vi "Main.Get Compiled Settings.vi"(8 "error in (no error)":errorcluster, 11 "Item Ref in":T1 format="%.0x") -> (0 "error out":errorcluster, 3 "Compiled":T2 {"Nodes"."Monitor"."Network"."Name" format="%.0x"; "Nodes"."Sim"."Network"."Name" format="%.0x"; "XNET"."Termination" items=["Off", "On"]})   [LabVIEW 2019, in "J1939 Addon Engine.lvlib"]
uses:
  J1939 Addon Engine.lvlib
  Addon Shared/Types/Compile Addon Settings.ctl
  Addon Shared/Types/XNET Settings.ctl
  Addon Shared/Types/SysDef FPGA Settings.ctl
  Addon Shared/Types/Compiled.Node Settings.ctl
  Addon Shared/Types/Compiled Monitor Tool Settings.ctl
  Addon Shared/Types/Monitor Settings.ctl
  Addon Shared/Types/Device Settings.ctl
  Addon Shared/Types/Incoming Settings.ctl
  Addon Shared/Types/Incoming Frame Settings.ctl
  <vilib>/NI VeriStand/Custom Device API/Block Data Reference.ctl
  <vilib>/NI VeriStand/Custom Device API/Data Reference.ctl
  Addon Shared/Types/Outgoing Settings.ctl
  Addon Shared/Types/Outgoing Frame Settings.ctl
  Addon Shared/Types/Outgoing Event Trigger Types.ctl
  SubModules/Frame-Protection-Support/Source/Shared/Types/Exported Frame Settings.ctl
  SubModules/Frame-Protection-Support/Source/Shared/Types/Exported Frame Type.ctl
  SubModules/Frame-Protection-Support/Source/Shared/Types/Exported Protection Settings.ctl
  SubModules/Frame-Protection-Support/Source/Shared/Types/Protection Type.ctl
  SubModules/Frame-Protection-Support/Source/Shared/Types/XNET Signal Configuration.ctl
  SubModules/Frame-Protection-Support/Source/Shared/Types/Exported Counter Settings.ctl
  SubModules/Frame-Protection-Support/Source/Shared/Types/Exported Event Trigger Type.ctl
  Addon Shared/Types/Complied Simulated Device Settings.ctl
  Addon Shared/Types/Compiled Simulated Settings.ctl
  <vilib>/NI VeriStand/Custom Device API/Custom Device Item Ref.ctl
  Addon Shared/SubVIs/Constants.vi
  <vilib>/NI VeriStand/Custom Device API/Get Item Property (Variant).vi
  <vilib>/NI VeriStand/Custom Device API/Custom Device API.lvlib
  Addon Shared/J1939 Addon Shared.lvlib
  SubModules/Frame-Protection-Support/Source/Shared/Protection and Counter Support Shared.lvlib
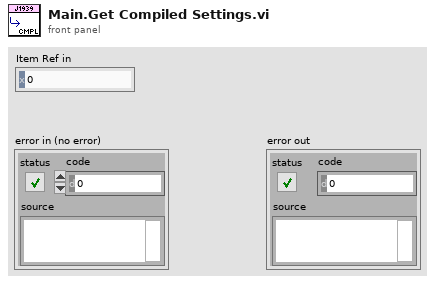
[diagram p1: front panel]
types:
  T1 = typedef "Custom Device API.lvlib/Custom Device Item Ref.ctl" = u64
  T2 = typedef "J1939 Addon Shared.lvlib/Compile Addon Settings.ctl" = cluster{"XNET":T3, "Bitfile":T4, "Nodes":T5, "Name":string}
  T3 = typedef "J1939 Addon Shared.lvlib/XNET Settings.ctl" = cluster{"Database":refnum<k21>, "Cluster":refnum<k21>, "Port":string, "Baud rate [Bd]":u32, "Termination":u32, "Incoming Decimation":u32, "Outgoing Decimation":u32}
  T4 = typedef "J1939 Addon Shared.lvlib/SysDef FPGA Settings.ctl" = cluster{"RT Path":path, "RIO Device":string, "Enable":bool}
  T5 = typedef "J1939 Addon Shared.lvlib/Compiled.Node Settings.ctl" = cluster{"Monitor":T6, "Sim":T23[]}
  T6 = typedef "J1939 Addon Shared.lvlib/Compiled Monitor Tool Settings.ctl" = cluster{"Network":T7, "Data":T8}
  T7 = typedef "J1939 Addon Shared.lvlib/Monitor Settings.ctl" = cluster{"Address":u8, "Name":u64, "Include DA":bool}
  T8 = typedef "J1939 Addon Shared.lvlib/Device Settings.ctl" = cluster{"Incoming":T9, "Outgoing":T13}
  T9 = typedef "J1939 Addon Shared.lvlib/Incoming Settings.ctl" = cluster{"Signals":string[], "Frames":T10[], "Data.Refs":T11[], "Data.Values":dbl[], "Timing.Use":bool, "Timing.Refs":T11[], "Timing.Values":dbl[], "Timing.Index":i32[]}
  T10 = typedef "J1939 Addon Shared.lvlib/Incoming Frame Settings.ctl" = cluster{"Signals":string[], "PGN":u32}
  T11 = typedef "Custom Device API.lvlib/Block Data Reference.ctl" = cluster{"Data Reference":T12, "Offset":u64, "Length":u64}
  T12 = typedef "Custom Device API.lvlib/Data Reference.ctl" = i32
  T13 = typedef "J1939 Addon Shared.lvlib/Outgoing Settings.ctl" = cluster{"Frames":T14[], "Data.Refs":T11[], "Data.Values":dbl[], "Disable.Refs":T11[], "Disable.Values":dbl[], "Trigger.Refs":T11[], "Trigger.Values":dbl[], "Frames.CountersAndProtections":T16[]}
  T14 = typedef "J1939 Addon Shared.lvlib/Outgoing Frame Settings.ctl" = cluster{"Signals":string[], "Channel Array Position":cluster{"Offset":u32, "Length":u32}, "PGN":u32, "Cyclic?":bool, "Disable?":bool, "Disable.Index":i32, "Trigger":T15, "Trigger.Index":i32}
  T15 = typedef "J1939 Addon Shared.lvlib/Outgoing Event Trigger Types.ctl" = enum16{"Channel value change", "Trigger channel (not zero)", "Channel value change or trigger channel (not zero)", "Trigger channel (any value change)", "Channel value change or trigger channel (any value change)"}
  T16 = typedef "Protection and Counter Support Shared.lvlib/Exported Frame Settings.ctl" = cluster{"Type":T17, "Frame ID":u32, "Payload Length":u32, "Signal XNET Paths":string[], "Frame.PrevData":dbl[], "VS Offset":i32, "VS Length":i32, "Generation Period":u32, "Has Protection?":bool, "Protection Configurations":T18[], "Has Counter":bool, "Counter Configurations":T21[], "Has Disable?":bool, "Disable VS Index":i32, "Transmit Trigger":T22, "Trigger VS Index":i32}
  T17 = typedef "Protection and Counter Support Shared.lvlib/Exported Frame Type.ctl" = enum16{"Periodic", "Event", "Periodic/Event"}
  T18 = typedef "Protection and Counter Support Shared.lvlib/Exported Protection Settings.ctl" = cluster{"Protection Frame Index":i32, "Protection Type":T19, "Data Indeces":i32[], "Initialized Data Array":dbl[], "Protection Signal XNET Paths":string[], "CRC Channels":T20[], "Protection VS Update Index":i32}
  T19 = typedef "Protection and Counter Support Shared.lvlib/Protection Type.ctl" = enum16{"Arb ID + Bytes Checksum with Inversion", "Arb ID + Bytes CRC with Inversion", "Reversed Raw Signal Checksum with Inversion", "Concatenated Two's Compliment"}
  T20 = typedef "Protection and Counter Support Shared.lvlib/XNET Signal Configuration.ctl" = cluster{"Start Bit":i32, "Name":string, "Number of bits":i32, "Scale":dbl, "Offset":dbl, "Data Type":u32, "Counter":bool}
  T21 = typedef "Protection and Counter Support Shared.lvlib/Exported Counter Settings.ctl" = cluster{"Frame Index":i32, "Max Count":dbl, "VS Index":i32, "Bit Length":i64}
  T22 = typedef "Protection and Counter Support Shared.lvlib/Exported Event Trigger Type.ctl" = enum16{"Channel value change", "Trigger channel (not zero)", "Channel value change or trigger channel (not zero)", "Trigger channel (any value change)", "Channel value change or trigger channel (any value change)"}
  T23 = typedef "J1939 Addon Shared.lvlib/Complied Simulated Device Settings.ctl" = cluster{"Network":T7, "Data":T8, "DTCs":T24}
  T24 = typedef "J1939 Addon Shared.lvlib/Compiled Simulated Settings.ctl" = cluster{"DM1.Ref":T11[], "DM1.Value":dbl[], "DM1.Enable.Ref":T11[], "DM1.Enable.Value":dbl[], "DM2.Ref":T11[], "DM2.Value":dbl[], "DM2.Enable.Ref":T11[], "DM2.Enable.Value":dbl[]}
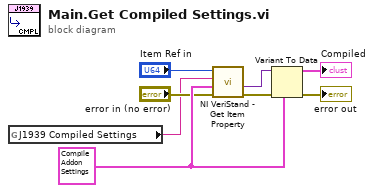
[diagram p0: block diagram]
diagram:
  w5 = T2 {"XNET"={"Database"="", "Cluster"="", "Port"="", "Baud rate [Bd]"=0, "Termination"=0, "Incoming Decimation"=0, "Outgoing Decimation"=0}, "Bitfile"={"RT Path"=path "", "RIO Device"="", "Enable"=FALSE}, "Nodes"={"Monitor"={"Network"={"Address"=0, "Name"=0, "Include DA"=FALSE}, "Data"={"Incoming"={"Signals"=[], "Frames"=[], "Data.Refs"=[], "Data.Values"=[], "Timing.Use"=FALSE, "Timing.Refs"=[], "Timing.Values"=[], "Timing.Index"=[]}, "Outgoing"={"Frames"=[], "Data.Refs"=[], "Data.Values"=[], "Disable.Refs"=[], "Disable.Values"=[], "Trigger.Refs"=[], "Trigger.Values"=[], "Frames.CountersAndProtections"=[]}}}, "Sim"=[]}, "Name"=""}
  n1 = global read "Constants.vi" "J1939 Compiled Settings"() -> (w3:string)
  n2 = call-poly <vilib>:"NI VeriStand - Get Item Property.vi"("error in (no error)"="error in (no error)", "Default Value"=w5, "Property Name"=w3, "Item Ref in"="Item Ref in") -> ("error out"=w2:errorcluster, "Value"=w1:variant)  [unwired: 4 in, 2 out]
  n3 = Variant To Data(error in=w2, type=w5, Variant=w1) -> (data=→"Compiled":T2, error out=→"error out":errorcluster)
